vi "input.vi"(8 "error in":errorcluster, 10 "data table in":T1, 11 "Scan Engine runtime in":refnum<class "Scan Engine runtime.lvclass">) -> (0 "error out":errorcluster, 2 "data table out":T1, 3 "Scan Engine runtime out":refnum<class "Scan Engine runtime.lvclass">)   [LabVIEW 2013, in "Scan Engine runtime.lvclass"]
doc: "Provides an interface for reading data from a module at runtime. While this interface performs no operations, a child should provide an override which may read from any open sessions, references, or interfaces."
uses:
  Scan Engine runtime.lvclass
  <vilib>/NI/Tag Bus/table/data table.ctl
  Scan Engine runtime.lvclass/Scan Engine runtime.ctl
  <vilib>/NI/Tag Bus/table/data polymorphs/write one/write Double.vi
  <vilib>/NI/Tag Bus/table/data polymorphs/write one/write Single.vi
  <vilib>/NI/Tag Bus/table/data polymorphs/write one/write I64.vi
  <vilib>/NI/Tag Bus/table/data polymorphs/write one/write I32.vi
  <vilib>/NI/Tag Bus/table/data polymorphs/write one/write I16.vi
  <vilib>/NI/Tag Bus/table/data polymorphs/write one/write I8.vi
  <vilib>/NI/Tag Bus/table/data polymorphs/write one/write U64.vi
  <vilib>/NI/Tag Bus/table/data polymorphs/write one/write U32.vi
  <vilib>/NI/Tag Bus/table/data polymorphs/write one/write U16.vi
  <vilib>/NI/Tag Bus/table/data polymorphs/write one/write U8.vi
  <vilib>/NI/Tag Bus/table/data polymorphs/write one/write Boolean.vi
  <vilib>/NI/Tag Bus/table/data table.lvlib
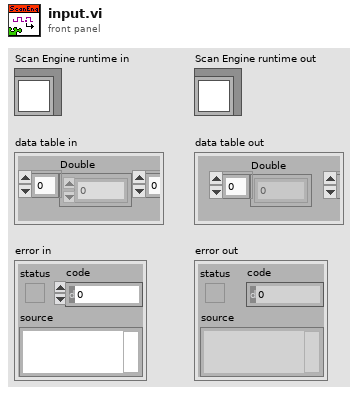
[diagram p1: front panel]
types:
  T1 = typedef "tag bus.lvlib/data table.lvlib/data table.ctl" = cluster{"Double":dbl[], "Single":sgl[], "I64":i64[], "I32":i32[], "I16":i16[], "I8":i8[], "U64":u64[], "U32":u32[], "U16":u16[], "U8":u8[], "Boolean":bool[], "String":string[], "Array of Double":cluster{"DBL Array":dbl[]}[], "Array of Single":cluster{"SGL Array":sgl[]}[], "Array of I64":cluster{"I64 Array":i64[]}[], "Array of I32":cluster{"I32 Array":i32[]}[], "Array of I16":cluster{"I16 Array":i16[]}[], "Array of I8":cluster{"I8 Array":i8[]}[], "Array of U64":cluster{"U64 Array":u64[]}[], "Array of U32":cluster{"U32 Array":u32[]}[], "Array of U16":cluster{"U16 Array":u16[]}[], "Array of U8":cluster{"U8 Array":u8[]}[], "Array of Boolean":cluster{"Boolean Array":bool[]}[], "Array of String":cluster{"String Array":string[]}[]}
  T2 = typedef "Scan Engine runtime.lvclass/Index Map.ctl" = cluster{"data type":T3, "variable ref":refnum<k21>, "index":i32}
  T3 = typedef "tag bus.lvlib/tag descriptor.lvclass/Data Type.ctl" = enum16{"Double", "Single", "I64", "I32", "I16", "I8", "U64", "U32", "U16", "U8", "Boolean", "String", "Array of Double", "Array of Single", "Array of I64", "Array of I32", "Array of I16", "Array of I8", "Array of U64", "Array of U32", "Array of U16", "Array of U8", "Array of Boolean", "Array of String"}
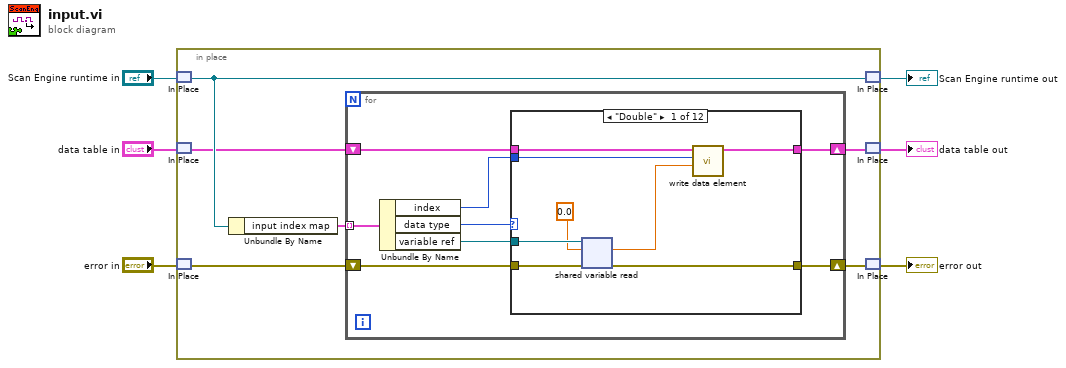
[diagram p0: block diagram]
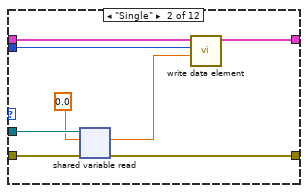
[diagram p2: hidden frame]
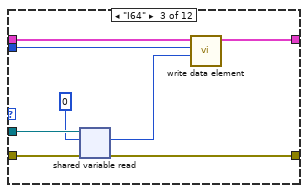
[diagram p3: hidden frame]
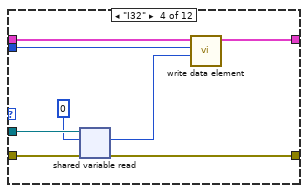
[diagram p4: hidden frame]
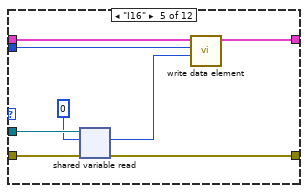
[diagram p5: hidden frame]
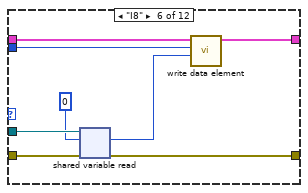
[diagram p6: hidden frame]
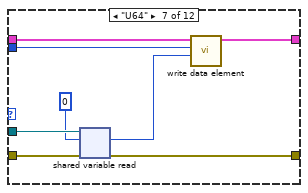
[diagram p7: hidden frame]
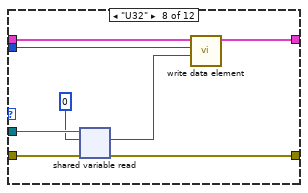
[diagram p8: hidden frame]
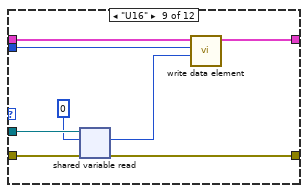
[diagram p9: hidden frame]
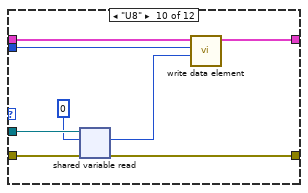
[diagram p10: hidden frame]
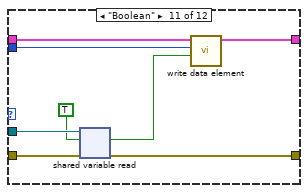
[diagram p11: hidden frame]
diagram:
  n1 = in-place {
    n2 = in-place-match #1("Scan Engine runtime in") -> (w12:refnum<class "Scan Engine runtime.lvclass">)
    n3 = in-place-match #2("data table in") -> (w11:T1)
    n4 = in-place-match #3("error in") -> (w9:errorcluster)
    n5 = Unbundle By Name(w12) -> ("input index map"=w7:T2[])
    n6 = for {
      shift-right: [w17] -> w10
      shift-left: w11 -> [w18]
      shift-right: [w13] -> w8
      shift-left: w9 -> [w14]
      tunnel: w7 -> [w20] mode=indexing
      n7 = Unbundle By Name(w20) -> ("index"=w16:i32, "data type"=w19:T3, "variable ref"=w15:refnum<k21>)
      n8 = case shown="\"Double\"" w19 {
        tunnel: w18 -> [w28 w36 w44 w52 w60 w68 w76 w84 w92 w100 w108 w110]
        tunnel: [w27 w35 w43 w51 w59 w67 w75 w83 w91 w99 w107 w110] -> w17
        tunnel: w16 -> [w26 w34 w42 w50 w58 w66 w74 w82 w90 w98 w106 _]
        tunnel: w15 -> [w25 w33 w41 w49 w57 w65 w73 w81 w89 w97 w105 _]
        tunnel: w14 -> [w24 w32 w40 w48 w56 w64 w72 w80 w88 w96 w104 w109]
        tunnel: [w22 w30 w38 w45 w53 w62 w70 w78 w85 w93 w102 w109] -> w13
        frame "Double" {
          n9 = shared-variable-read(w25, w24, 0.0) -> (w22:errorcluster, w23:dbl)  [unwired: 1 out]
          n10 = call-poly <vilib>:"write data element.vi"("value"=w23, "index"=w26, "data table in"=w28) -> ("data table out"=w27:T1)  [unwired: 8 in]
        }
        frame "Single" {
          n11 = shared-variable-read(w33, w32, sgl 0.0) -> (w30:errorcluster, w31:sgl)  [unwired: 1 out]
          n12 = call-poly <vilib>:"write data element.vi"("value"=w31, "index"=w34, "data table in"=w36) -> ("data table out"=w35:T1)  [unwired: 8 in]
        }
        frame "I64" {
          n13 = shared-variable-read(w41, w40, i64 0) -> (w38:errorcluster, w39:i64)  [unwired: 1 out]
          n14 = call-poly <vilib>:"write data element.vi"("value"=w39, "index"=w42, "data table in"=w44) -> ("data table out"=w43:T1)  [unwired: 8 in]
        }
        frame "I32" {
          n15 = shared-variable-read(w49, w48, 0) -> (w45:errorcluster, w46:i32)  [unwired: 1 out]
          n16 = call-poly <vilib>:"write data element.vi"("value"=w46, "index"=w50, "data table in"=w52) -> ("data table out"=w51:T1)  [unwired: 8 in]
        }
        frame "I16" {
          n17 = shared-variable-read(w57, w56, i16 0) -> (w53:errorcluster, w54:i16)  [unwired: 1 out]
          n18 = call-poly <vilib>:"write data element.vi"("value"=w54, "index"=w58, "data table in"=w60) -> ("data table out"=w59:T1)  [unwired: 8 in]
        }
        frame "I8" {
          n19 = shared-variable-read(w65, w64, i8 0) -> (w62:errorcluster, w63:i8)  [unwired: 1 out]
          n20 = call-poly <vilib>:"write data element.vi"("value"=w63, "index"=w66, "data table in"=w68) -> ("data table out"=w67:T1)  [unwired: 8 in]
        }
        frame "U64" {
          n21 = shared-variable-read(w73, w72, u64 0) -> (w70:errorcluster, w71:u64)  [unwired: 1 out]
          n22 = call-poly <vilib>:"write data element.vi"("value"=w71, "index"=w74, "data table in"=w76) -> ("data table out"=w75:T1)  [unwired: 8 in]
        }
        frame "U32" {
          n23 = shared-variable-read(w81, w80, u32 0) -> (w78:errorcluster, w79:u32)  [unwired: 1 out]
          n24 = call-poly <vilib>:"write data element.vi"("value"=w79, "index"=w82, "data table in"=w84) -> ("data table out"=w83:T1)  [unwired: 8 in]
        }
        frame "U16" {
          n25 = shared-variable-read(w89, w88, u16 0) -> (w85:errorcluster, w86:u16)  [unwired: 1 out]
          n26 = call-poly <vilib>:"write data element.vi"("value"=w86, "index"=w90, "data table in"=w92) -> ("data table out"=w91:T1)  [unwired: 8 in]
        }
        frame "U8" {
          n27 = shared-variable-read(w97, w96, u8 0) -> (w93:errorcluster, w94:u8)  [unwired: 1 out]
          n28 = call-poly <vilib>:"write data element.vi"("value"=w94, "index"=w98, "data table in"=w100) -> ("data table out"=w99:T1)  [unwired: 8 in]
        }
        frame "Boolean" {
          n29 = shared-variable-read(w105, w104, TRUE) -> (w102:errorcluster, w103:bool)  [unwired: 1 out]
          n30 = call-poly <vilib>:"write data element.vi"("value"=w103, "index"=w106, "data table in"=w108) -> ("data table out"=w107:T1)  [unwired: 8 in]
        }
        frame Default {
        }
      }
    }
    n31 = in-place-match #1(w12) -> (→"Scan Engine runtime out":refnum<class "Scan Engine runtime.lvclass">)
    n32 = in-place-match #2(w10) -> (→"data table out":T1)
    n33 = in-place-match #3(w8) -> (→"error out":errorcluster)
  }
